vi "Main_Steuerung.vi"() -> ()   [LabVIEW 2016]
uses:
  <vilib>/rvi/interface/nirviReadWriteControl/nirviReadWriteControl.xnode
  NiFpgaLv.dll
  <vilib>/Utility/error.llb/Error Cluster From Error Code.vi
  <vilib>/rvi/interface/Simulation/niFpgaSimulationCallBeginRW.vi
  <vilib>/rvi/errors/niLvFpgaAdjustHostInterfaceError.vi
  <vilib>/rvi/interface/nirviOpenFPGA/nirviOpenFPGA.xnode
  <vilib>/rvi/interface/nirviMethod/nirviMethod.xnode
  <vilib>/FPGAPlugInAG/Dynamic/niLvFpga_Reset_Dynamic.vi
  <vilib>/FPGAPlugInAG/Dynamic/niLvFpga_Run_Dynamic.vi
  <vilib>/rvi/interface/nirviCloseFPGA/nirviCloseFPGA.xnode
  <vilib>/FPGAPlugInAG/Dynamic/niLvFpga_Abort_Dynamic.vi
  <vilib>/ptbypt/NI_PtbyPt.lvlib
  <vilib>/Analysis/NI_AALBase.lvlib
  <vilib>/Analysis/1siggen.llb/Ramp Pattern by Samples.vi
  <vilib>/regexp/Match Regular Expression.xnode
  <vilib>/FPGAPlugInAG/Dynamic/niLvFpga_Close_Dynamic.vi
  <vilib>/rvi/interface/common/dynamic/niFpgaDynamicAddResources.vi
  FPGA Bitfiles/AKZ1_FPGATarget_MainFPGA_-zWm+JuPuU4.lvbitx
  Main_FPGA.vi
  <vilib>/FPGAPlugInAG/cRIO-9082/niLvFpga_Open_cRIO-9082.vi
  FPGA Bitfiles/AKZ1_FPGATarget3_EncoderPosition&_wC3QGglG6Rs.lvbitx
  FPGA VIs/Encoder Position & Velocity (FPGA).vi
  <vilib>/FPGAPlugInAG/NI 9154/niLvFpga_Open_NI 9154.vi
panel:
  in  "Output Range Bremse L":T1={"output high"=10.0, "output low"=-10.0}
  in  "Output Range Bremse R":T1={"output high"=10.0, "output low"=-10.0}
  in  "Stop":bool
  in  "Systemreset / ON":bool
  out "Alarme":T2
  in  "Alarme On":T3={"A 1"=TRUE, "A 2"=TRUE, "A 3"=FALSE, "A 4"=TRUE, "A 5"=TRUE, "A 6"=TRUE, "A 7"=TRUE, "A 8"=TRUE, "A 9"=TRUE, "A 10"=TRUE, "A 11"=TRUE, "A 12"=TRUE, "A 13"=TRUE, "A 14"=TRUE, "A 15"=TRUE, "A 16"=TRUE, "A 17"=FALSE, "A 18"=FALSE, "A 19"=FALSE, "A 20"=FALSE, "A 21"=FALSE, "A 22"=FALSE, "A 23"=FALSE, "A 24"=FALSE}
  in  "Masteralarm On":bool
  out "Masteralarm":bool
  in  "PID gains Bremse L":T4={"proportional gain (Kc)"=5.0, "integral gain (Kc*Ts/Ti)"=0.1015625, "derivative gain (Kc*Td/Ts)"=0.0}
  in  "PID gains Bremse R":T4={"proportional gain (Kc)"=5.0, "integral gain (Kc*Ts/Ti)"=0.1015625, "derivative gain (Kc*Td/Ts)"=0.0}
  in  "PID gains Bremse H":T4={"proportional gain (Kc)"=5.0, "integral gain (Kc*Ts/Ti)"=0.1015625, "derivative gain (Kc*Td/Ts)"=0.0}
  in  "PID gains Fahrhebelsteller":T4={"proportional gain (Kc)"=1.5, "integral gain (Kc*Ts/Ti)"=0.1015625, "derivative gain (Kc*Td/Ts)"=0.0}
  out "Recht":dbl(knob) scale=-10.0..10.0
  out "Link":dbl(knob) scale=-10.0..10.0
  out "L":dbl
  out "R":dbl
  in  "Rampe Down":u32=5
  in  "Count (mSec) Rampe H":u32=2
  in  "Count (mSec) H":u32=10
  out "output Rampe H":dbl
  in  "milliseconds to wait Rampe H":u32=10
  in  "type Rampe H":u16(ring) items=["Linear", "Logarithmic"]
  in  "sample length H":i32=100
  in  "milliseconds to wait Fahrhebel":u32=10
  in  "type Fahrhebel":u16(ring) items=["Linear", "Logarithmic"]
  out "output Fahrhebel":dbl
  in  "Count (mSec) Fahrhebel":u32=22
  in  "sample length LR":i32=100
  in  "sample length DM":i32=100
  in  "Count (mSec) Normal LR":u32=10
  in  "type Rampe LR":u16(ring) items=["Linear", "Logarithmic"]
  out "output Rampe LR":dbl format="%.2f"
  in  "milliseconds to wait Rampe LR":u32=10
  in  "Count (mSec) Rampe LR":u32=2
  in  "error in (no error)":errorcluster
  out "Punktenanzahl":i32
  out "Punktentabelle":dbl[][](array[numeric])
  out "error out":errorcluster
  in  "Tab Control":enum32{"H", "L-R", "H-L-R", "System"}(tab)
  in  "PID Out H":bool=TRUE
  in  "Rout H":bool
  out "Wellendrehmoment mit Übersetzung  H":dbl(knob) scale=-2000.0..2000.0
  out "Drehmoment Hinten":dbl(knob) scale=-2000.0..2000.0
  out "Drehzahl Hinten":dbl(knob) scale=0.0..8000.0
  in  "Bremse\nFrei H":bool
  in  "Reset / On\n H":bool
  in  "Steuerung\nOn H":bool
  in  "Lüftung\nOn H":bool
  out "Meldungen H":T5
  in  "Wellendrehzahl\n Soll H":dbl(slide) scale=-8000.0..8000.0
  out "Wellendrehzahl mit Übersetzung H":dbl(knob) scale=0.0..12000.0
  in  "Übersetzung H":dbl=3.15
  in  "Start Rampe H":dbl=900.0
  in  "Ende Rampe H":dbl=5100.0
  in  "Zeit (Sec) Rampe H":i32=30
  out "Rampe H Aktiv":bool
  in  "Rampe H Stop":bool
  in  "Rampe H Start":bool
  in  "Übersetzung H\nmit":bool=TRUE
  out "Rampe H  LED":bool
  out "Startwert Rampe LR 2":dbl format="%#_3f"
  in  "Wellen\nmoment\n Soll H":dbl(slide) scale=-2000.0..2000.0
  in  "Drehzahl/moment H":bool
  in  "Rampe H Runter":bool
  in  "PID Out LR":bool=TRUE
  out "Startwert Rampe LR":dbl format="%#_3f"
  out "Rampe LR  LED":bool
  in  "Übersetzung LR\nmit":bool=TRUE
  out "Abweichung":dbl(knob) scale=-30.0..30.0
  in  "Wellen\nmoment\n Soll LR":dbl(slide) scale=-2000.0..2000.0
  in  "Drehzahl/moment LR":bool
  out "Wellendrehmoment mit Übersetzung":dbl(knob) scale=-400.0..400.0
  out "Drehmoment Rechts":dbl(knob) scale=-2000.0..2000.0
  out "Drehmoment Links":dbl(knob) scale=-2000.0..2000.0
  out "Drehzahl Rechts":dbl(knob) scale=-3000.0..3000.0
  out "Drehzahl Links":dbl(knob) scale=-3000.0..3000.0
  in  "Bremse\nFrei":bool
  in  "Reset / On":bool
  in  "Steuerung\nOn":bool
  in  "Lüftung\nOn":bool
  out "Meldungen L-R":T6
  in  "Wellen\ndrehzahl\n Soll":dbl(slide) scale=-3000.0..3000.0 scale format="%4d"
  out "Wellendrehzahl mit Übersetzung":dbl(knob) scale=0.0..5000.0
  in  "Übersetzung LR":dbl=3.88
  in  "Rampe LR Start":bool
  in  "Rampe LR Runter":bool
  in  "Rampe LR Stop":bool
  out "Rampe LR Aktiv":bool
  in  "Zeit (Sec) Rampe LR":i32=60
  in  "Ende Rampe LR":dbl=4800.0
  in  "Start Rampe LR":dbl=880.0
  in  "Rout LR":bool
  in  "Tab Control 2":enum32{"Benzinmotor", "Elektromototr"}(tab)
  out "Rampe Fahrregler  LED":bool
  in  "Fahrregler Runter":bool
  in  "Fahrregler Stop":bool
  out "Fahrregler Aktiv":bool
  in  "Fahrregler Start":bool
  in  "PID Regler Fahrhebel\nWellenmoment Soll":bool
  in  "Motor\nStart":bool
  in  "Vorglühen\nOn":bool
  in  "Zündung\nOn":bool
  in  "Kraftstoff\nOn":bool
  out "Fahrhebelsteller":u8(slide) scale=0.0..100.0
  in  "Fahrhebelsteller Soll":dbl(slide) scale=0.0..100.0
  in  "Freigabe Fahrhebel":bool
  in  "Kupplung\nOffen":bool=TRUE
  out "Kupplung":cluster{"Offen":bool, "Geschlossen":bool}
  in  "Zeit (Sec) Fahrregler":i32=20
  in  "Ende Fahrregler":dbl=100.0
  in  "Start Fahrregler":dbl
  in  "Kennfeld Wellenmoment laden\nx,xx Prozent einstellen":bool
  in  "Prozent":dbl=0.5
  in  "Temperaturregelung\nFreigabe":bool
  in  "Temperaturregelung\nWait":bool
  out "Höhe M":fxp<+/-,24,5> format="%#.2g"
  out "Endlage Unten M":bool
  out "Endlage Oben M":bool
  out "Oben M":bool
  out "Unten M":bool
  in  "Freigabe Höhe M":bool
  in  "Richtung Höhe M":bool
  in  "Freigabe Drehzahl M":bool
  in  "Richtung Drehzahl M":bool
  in  "Freigabe Bremse M":bool
  in  "Run Button":bool
  in  "Hydraulikpumpensteller":dbl=11.0
  in  "Manual":bool
  in  "Up Button":bool
  in  "Down Button":bool
  in  "RPMK":dbl=300.0
  in  "Drehmoment Motor":dbl
  in  "Hydraulikkupplung":dbl
  # "ohne"
  # "ohne"
  # "Links"
  # "Rechts"
  # "System nicht bereit!"
  # "Geschlossen"
  # "%"
  # "%"
  # "%"
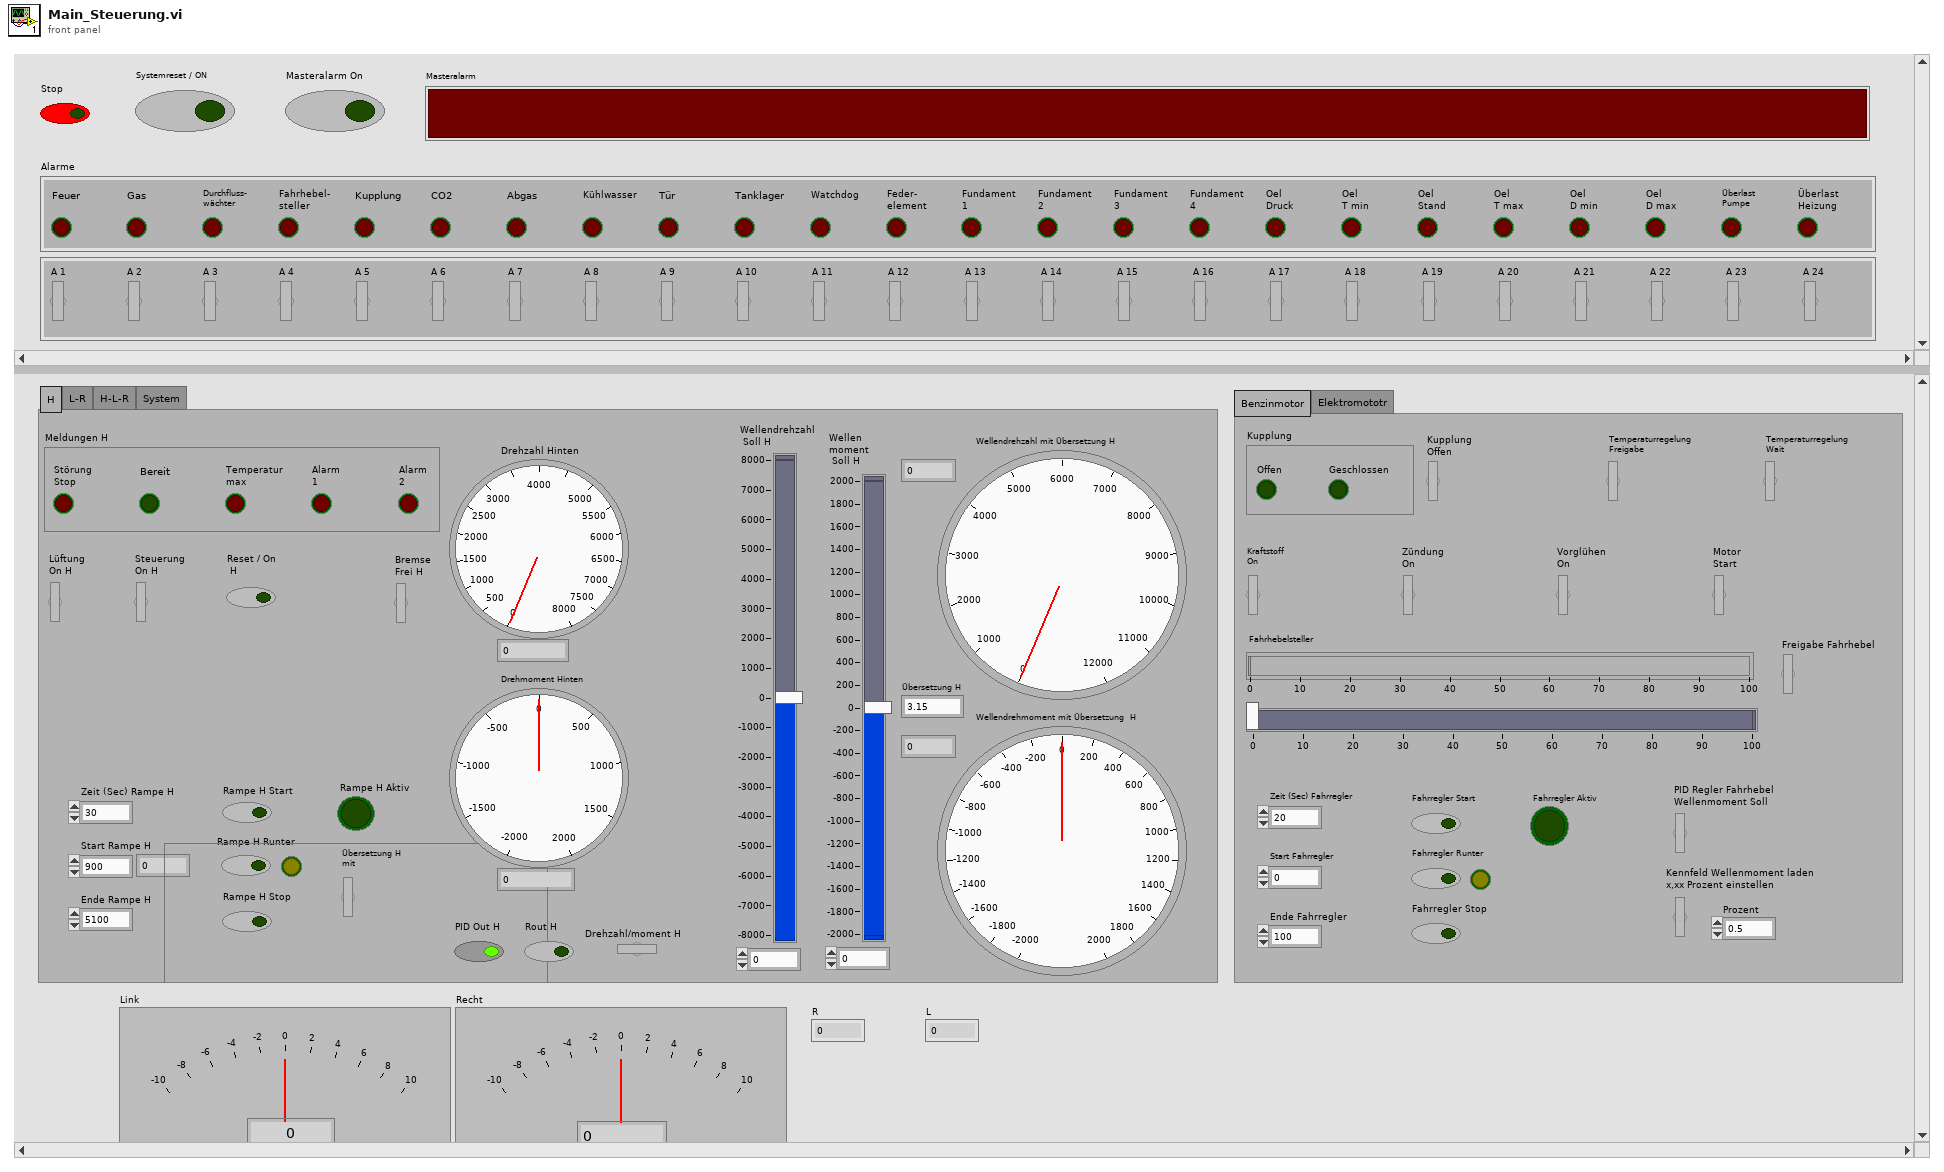
[diagram p1: front panel]
types:
  T1 = cluster{"output high":fxp<+/-,16,5>, "output low":fxp<+/-,16,5>}
  T2 = cluster{"Feuer\n":bool, "Gas\n":bool, "Durchfluss-\nwächter":bool, "Fahrhebel-\nsteller":bool, "Kupplung\n":bool, "CO2\n":bool, "Abgas\n":bool, "Kühlwasser\n":bool, "Tür\n":bool, "Tanklager\n":bool, "Watchdog\n":bool, "Feder-\nelement":bool, "Fundament\n1":bool, "Fundament\n2":bool, "Fundament\n3":bool, "Fundament\n4":bool, "Oel\nDruck":bool, "Oel\nT min":bool, "Oel\nStand":bool, "Oel\nT max":bool, "Oel\nD min":bool, "Oel\nD max":bool, "Überlast\nPumpe":bool, "Überlast\nHeizung":bool}
  T3 = cluster{"A 1":bool, "A 2":bool, "A 3":bool, "A 4":bool, "A 5":bool, "A 6":bool, "A 7":bool, "A 8":bool, "A 9":bool, "A 10":bool, "A 11":bool, "A 12":bool, "A 13":bool, "A 14":bool, "A 15":bool, "A 16":bool, "A 17":bool, "A 18":bool, "A 19":bool, "A 20":bool, "A 21":bool, "A 22":bool, "A 23":bool, "A 24":bool}
  T4 = cluster{"proportional gain (Kc)":fxp<+/-,16,8>, "integral gain (Kc*Ts/Ti)":fxp<+/-,16,8>, "derivative gain (Kc*Td/Ts)":fxp<+/-,16,8>}
  T5 = cluster{"Störung\nStop":bool, "Bereit\n":bool, "Temperatur\nmax":bool, "Alarm\n1":bool, "Alarm\n2":bool}
  T6 = cluster{"Störung\nStop":bool, "Bereit\n":bool, "Temperatur\nmax":bool, "Alarm\n1":bool, "Alarm\n2":bool, "Störung\nStop":bool, "Bereit\n":bool, "Temperatur\nmax":bool, "Alarm\n1":bool, "Alarm\n2":bool}
  T7 = enum16{"open", "replace", "create", "open or create", "replace or create", "replace or create with confirmation"}
  T8 = cluster{"Mod5/Alarm 1 Feuer":void, "Mod5/Alarm 2 Gas":bool, "Mod5/Alarm 3 Durchflusswächter":void, "Mod5/Alarm 4 Fahrhebelsteller":void, "Mod5/Alarm 5 Kupplung":void, "Mod5/Alarm 6 CO2":bool, "Mod5/Alarm 7 Abgas":void, "Mod5/Alarm 8 Kühlwasser":void, "Mod5/Alarm 9 Tür":void, "Mod5/Alarm 10 Tanklager":void, "Mod5/Alarm 11 Watchdog":bool, "Mod5/Alarm 12 Federelement":void, "Mod5/Alarm 13 Fundament 1":bool, "Mod5/Alarm 14 Fundament 2":bool, "Mod5/Alarm 15 Fundament 3":bool, "Mod5/Alarm 16 Fundament 4":bool, "Mod6/Alarm 17 Differnzdruck Öl":void, "Mod6/Alarm 19 Temperatur Min ÖL":void, "Mod6/Alarm 18 Nivau Öl":void, "Mod6/Alarm 20 Temperatur Max Öl":void, "Mod6/Alarm 21 Druck Min Öl":void, "Mod6/Alarm 22 Druck Max Öl":void, "Mod6/Alarm 23 Überlast Pumpe Öl":void, "Mod6/Alarm 24 Überlast Heizung Öl":void}
  T9 = cluster{"Mod5/Störung Bremse L":void, "Mod5/Bereit Bremse L":void, "Mod5/Temperatur Bremse L":void, "Mod5/Alarm 1 Bremse L":void, "Mod5/Alarm 2 Bremse L":void, "Mod5/Störung Bremse R":void, "Mod5/Bereit Bremse R":void, "Mod5/Temperatur Bremse R":void, "Mod5/Alarm 1 Bremse R":void, "Mod5/Alarm 2 Bremse R":void}
  T10 = cluster{"Mod6/Störung Bremse H":void, "Mod6/Bereit Bremse H":void, "Mod6/Temperatur Bremse H":void, "Mod6/Alarm 1 Bremse H":void, "Mod6/Alarm 2 Bremse H":void}
  T11 = cluster{"Mod6/Kupplung Zu":void, "Mod6/Kupplung Auf":void}
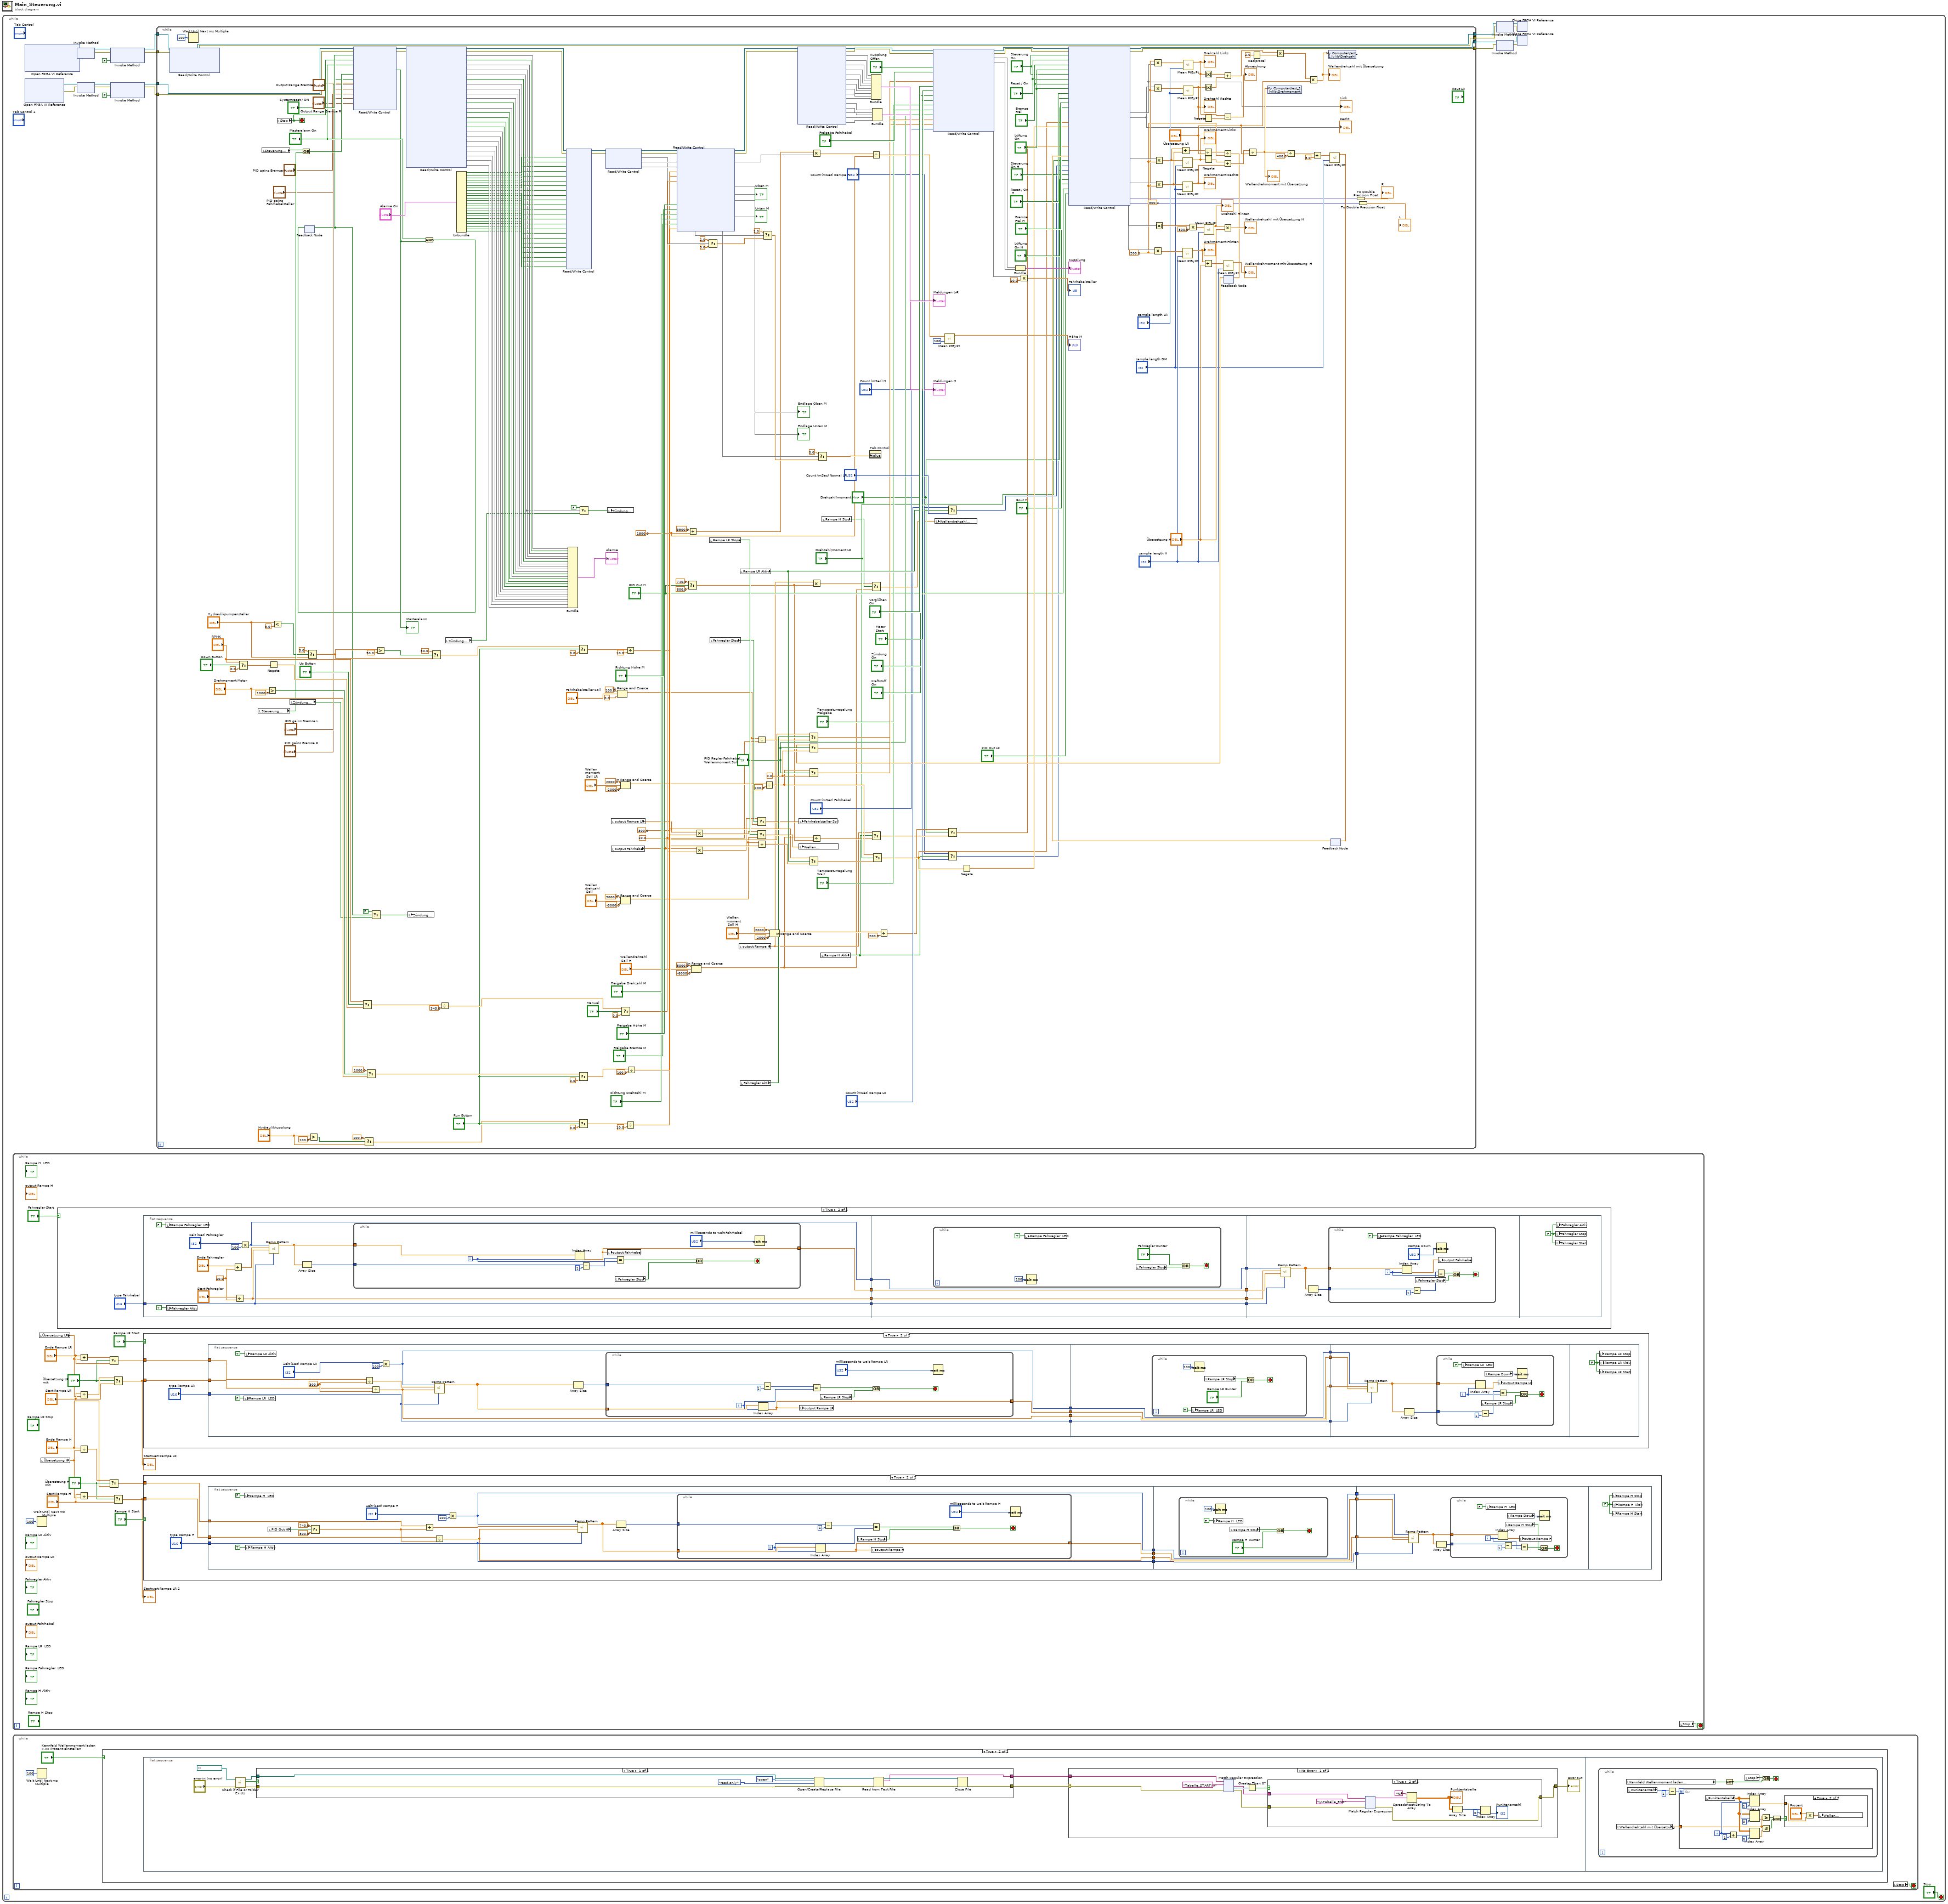
[diagram p0: block diagram]
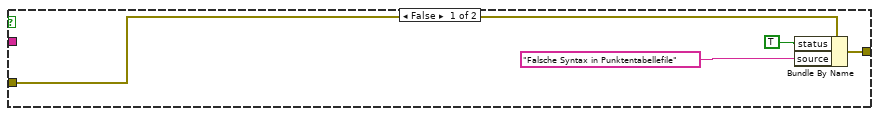
[diagram p3: hidden frame]
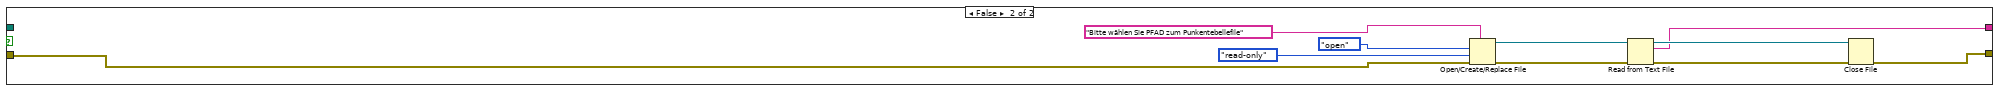
[diagram p5: hidden frame]
diagram:
  n1 = while {
    stop <- "Stop" stop-if-true
    n2 = while {
      stop <- w344 stop-if-true
      n3 = Wait Until Next ms Multiple(millisecond multiple=u32 100) -> ()  [unwired: 1 out]
      n4 = local read "Übersetzung LR"() -> (w336:dbl)
      n5 = local read "Übersetzung H"() -> (w328:dbl)
      n6 = case shown="True" "Fahrregler Start" {
        frame False {
        }
        frame True {
          n7 = flat-sequence {
            tunnel: "type Fahrhebel" -> [w426]
            tunnel: [w423] -> w418
            tunnel: [w426] -> w416
            tunnel: [w425] -> w414
            tunnel: [w424] -> w412
            tunnel: w418 -> [w447]
            tunnel: [w447] -> w417
            tunnel: w416 -> [w446]
            tunnel: [w446] -> w415
            tunnel: w414 -> [w445]
            tunnel: [w445] -> w413
            tunnel: w412 -> [w444]
            tunnel: [w444] -> w411
            tunnel: w417 -> [w458]
            tunnel: w415 -> [w457]
            tunnel: w413 -> [w456]
            tunnel: w411 -> [w455]
            frame #0 {
              w430 = 10.0 ("y")
              n8 = local write "Rampe Fahrregler  LED"(FALSE) -> ()
              n9 = local write "Fahrregler Aktiv"(TRUE) -> ()
              n10 = Divide(x="Ende Fahrregler", y=w430) -> (x/y=w432:dbl)
              n11 = Divide(x="Start Fahrregler", y=w430) -> (x/y=w424:dbl)
              n12 = Multiply(x="Zeit (Sec) Fahrregler", y=100) -> (x*y=w423:i32)
              n13 = call-poly <vilib>:"Ramp Pattern.vi"("type"=w426, "start"=w424, "end"=w432, "samples"=w423) -> ("Ramp Pattern"=w428:dbl[])  [unwired: 6 in, 1 out]
              n14 = Array Size(array=w428) -> (size(s)=w427:i32)
              n15 = while {
                tunnel: w428 -> [w443]
                tunnel: w427 -> [w442]
                tunnel: [w434] -> w425
                i -> [w439]
                stop <- w437 stop-if-true
                n16 = Index Array(array=w443, index=w439) -> (element=w434:dbl)
                n17 = Subtract(x=w442, y=1) -> (x-y=w440:i32)
                n18 = local write "output Fahrhebel"(w434) -> ()
                n19 = local read "Fahrregler Stop"() -> (w436:bool)
                n20 = Equal?(x=w440, y=w439) -> (x = y?=w438:bool)
                n21 = Or(x=w438, y=w436) -> (x .or. y?=w437:bool)
                n22 = Wait (ms)(milliseconds to wait="milliseconds to wait Fahrhebel") -> ()  [unwired: 1 out]
              }
            }
            frame #1 {
              n23 = while {
                stop <- w451 stop-if-true
                n24 = local write "Rampe Fahrregler  LED"(TRUE) -> ()
                n25 = Wait (ms)(milliseconds to wait=u32 100) -> ()  [unwired: 1 out]
                n26 = local read "Fahrregler Stop"() -> (w450:bool)
                n27 = Or(x="Fahrregler Runter", y=w450) -> (x .or. y?=w451:bool)
              }
            }
            frame #2 {
              n28 = call-poly <vilib>:"Ramp Pattern.vi"("type"=w457, "start"=w456, "end"=w455, "samples"=w458) -> ("Ramp Pattern"=w454:dbl[])  [unwired: 6 in, 1 out]
              n29 = Array Size(array=w454) -> (size(s)=w453:i32)
              n30 = while {
                tunnel: w454 -> [w469]
                tunnel: w453 -> [w468]
                i -> [w465]
                stop <- w463 stop-if-true
                n31 = local write "Rampe Fahrregler  LED"(FALSE) -> ()
                n32 = Index Array(array=w469, index=w465) -> (element=w461:dbl)
                n33 = Subtract(x=w468, y=1) -> (x-y=w466:i32)
                n34 = local read "Fahrregler Stop"() -> (w462:bool)
                n35 = Equal?(x=w466, y=w465) -> (x = y?=w464:bool)
                n36 = Wait (ms)(milliseconds to wait="Rampe Down") -> ()  [unwired: 1 out]
                n37 = local write "output Fahrhebel"(w461) -> ()
                n38 = Or(x=w464, y=w462) -> (x .or. y?=w463:bool)
              }
            }
            frame #3 {
              w470 = FALSE
              n39 = local write "Fahrregler Stop"(w470) -> ()
              n40 = local write "Fahrregler Start"(w470) -> ()
              n41 = local write "Fahrregler Aktiv"(w470) -> ()
            }
          }
        }
      }
      n42 = Divide(x="Ende Rampe LR", y=w336) -> (x/y=w341:dbl)
      n43 = Divide(x="Start Rampe LR", y=w336) -> (x/y=w339:dbl)
      n44 = Divide(x="Ende Rampe H", y=w328) -> (x/y=w332:dbl)
      n45 = Divide(x="Start Rampe H", y=w328) -> (x/y=w333:dbl)
      n46 = Select(t=w341, s="Übersetzung LR\nmit", f="Ende Rampe LR") -> (s? t:f=w342:dbl)
      n47 = Select(t=w332, s="Übersetzung H\nmit", f="Ende Rampe H") -> (s? t:f=w327:dbl)
      n48 = Select(t=w339, s="Übersetzung LR\nmit", f="Start Rampe LR") -> (s? t:f=w335:dbl)
      "Startwert Rampe LR" <- w335
      n49 = Select(t=w333, s="Übersetzung H\nmit", f="Start Rampe H") -> (s? t:f=w326:dbl)
      "Startwert Rampe LR 2" <- w326
      n50 = case shown="True" "Rampe LR Start" {
        tunnel: w335 -> [_ w472]
        tunnel: w342 -> [_ w471]
        frame False {
        }
        frame True {
          n51 = flat-sequence {
            tunnel: [w487] -> w480
            tunnel: [w492] -> w478
            tunnel: [w491] -> w476
            tunnel: [w489] -> w474
            tunnel: "type Rampe LR" -> [w489]
            tunnel: w472 -> [w482]
            tunnel: w471 -> [w483]
            tunnel: [w509] -> w481
            tunnel: w480 -> [w509]
            tunnel: [w508] -> w479
            tunnel: w478 -> [w508]
            tunnel: [w507] -> w477
            tunnel: w476 -> [w507]
            tunnel: [w506] -> w475
            tunnel: w474 -> [w506]
            tunnel: w481 -> [w520]
            tunnel: w479 -> [w519]
            tunnel: w477 -> [w518]
            tunnel: w475 -> [w517]
            frame #0 {
              w488 = 300.0
              n52 = local write "Rampe LR  LED"(FALSE) -> ()
              n53 = local write "Rampe LR Aktiv"(TRUE) -> ()
              n54 = Divide(x=w483, y=w488) -> (x/y=w493:dbl)
              n55 = Divide(x=w482, y=w488) -> (x/y=w492:dbl)
              n56 = Multiply(x="Zeit (Sec) Rampe LR", y=100) -> (x*y=w487:i32)
              n57 = call-poly <vilib>:"Ramp Pattern.vi"("type"=w489, "start"=w492, "end"=w493, "samples"=w487) -> ("Ramp Pattern"=w494:dbl[])  [unwired: 6 in, 1 out]
              n58 = Array Size(array=w494) -> (size(s)=w495:i32)
              n59 = while {
                tunnel: w494 -> [w505]
                tunnel: w495 -> [w504]
                tunnel: [w496] -> w491
                i -> [w501]
                stop <- w498 stop-if-true
                n60 = Index Array(array=w505, index=w501) -> (element=w496:dbl)
                n61 = Subtract(x=w504, y=1) -> (x-y=w502:i32)
                n62 = local write "output Rampe LR"(w496) -> ()
                n63 = Equal?(x=w502, y=w501) -> (x = y?=w500:bool)
                n64 = local read "Rampe LR Stop"() -> (w497:bool)
                n65 = Or(x=w500, y=w497) -> (x .or. y?=w498:bool)
                n66 = Wait (ms)(milliseconds to wait="milliseconds to wait Rampe LR") -> ()  [unwired: 1 out]
              }
            }
            frame #1 {
              n67 = while {
                stop <- w512 stop-if-true
                n68 = local write "Rampe LR  LED"(TRUE) -> ()
                n69 = Wait (ms)(milliseconds to wait=u32 100) -> ()  [unwired: 1 out]
                n70 = local read "Rampe LR Stop"() -> (w511:bool)
                n71 = Or(x=w511, y="Rampe LR Runter") -> (x .or. y?=w512:bool)
              }
            }
            frame #2 {
              n72 = call-poly <vilib>:"Ramp Pattern.vi"("type"=w517, "start"=w518, "end"=w519, "samples"=w520) -> ("Ramp Pattern"=w516:dbl[])  [unwired: 6 in, 1 out]
              n73 = Array Size(array=w516) -> (size(s)=w515:i32)
              n74 = while {
                tunnel: w516 -> [w531]
                tunnel: w515 -> [w530]
                i -> [w527]
                stop <- w525 stop-if-true
                n75 = local write "Rampe LR  LED"(FALSE) -> ()
                n76 = Index Array(array=w531, index=w527) -> (element=w523:dbl)
                n77 = Subtract(x=w530, y=1) -> (x-y=w528:i32)
                n78 = local read "Rampe LR Stop"() -> (w524:bool)
                n79 = local read "Rampe Down"() -> (w521:u32)
                n80 = local write "output Rampe LR"(w523) -> ()
                n81 = Equal?(x=w528, y=w527) -> (x = y?=w526:bool)
                n82 = Wait (ms)(milliseconds to wait=w521) -> ()  [unwired: 1 out]
                n83 = Or(x=w526, y=w524) -> (x .or. y?=w525:bool)
              }
            }
            frame #3 {
              w532 = FALSE
              n84 = local write "Rampe LR Stop"(w532) -> ()
              n85 = local write "Rampe LR Start"(w532) -> ()
              n86 = local write "Rampe LR Aktiv"(w532) -> ()
            }
          }
        }
      }
      n87 = case shown="True" "Rampe H Start" {
        tunnel: w327 -> [_ w356]
        tunnel: w326 -> [_ w355]
        frame False {
        }
        frame True {
          n88 = flat-sequence {
            tunnel: w356 -> [w370]
            tunnel: w355 -> [w369]
            tunnel: "type Rampe H" -> [w364]
            tunnel: [w364] -> w353
            tunnel: [w363] -> w351
            tunnel: [w362] -> w349
            tunnel: [w361] -> w347
            tunnel: w353 -> [w387]
            tunnel: [w387] -> w352
            tunnel: w351 -> [w386]
            tunnel: [w386] -> w350
            tunnel: w349 -> [w385]
            tunnel: [w385] -> w348
            tunnel: w347 -> [w384]
            tunnel: [w384] -> w346
            tunnel: w352 -> [w396]
            tunnel: w350 -> [w395]
            tunnel: w348 -> [w394]
            tunnel: w346 -> [w393]
            frame #0 {
              n89 = local write "Rampe H  LED"(FALSE ("Rampe H  LED")) -> ()
              n90 = local write "Rampe H Aktiv"(TRUE ("Rampe H Aktiv")) -> ()
              n91 = local read "PID Out H"() -> (w357:bool)
              n92 = Select(t=740.0, s=w357, f=800.0 ("y")) -> (s? t:f=w358:dbl)
              n93 = Divide(x=w370, y=w358) -> (x/y=w371:dbl)
              n94 = Divide(x=w369, y=w358) -> (x/y=w362:dbl)
              n95 = Multiply(x="Zeit (Sec) Rampe H", y=100) -> (x*y=w363:i32)
              n96 = call-poly <vilib>:"Ramp Pattern.vi"("type"=w364, "start"=w362, "end"=w371, "samples"=w363) -> ("Ramp Pattern"=w366:dbl[])  [unwired: 6 in, 1 out]
              n97 = Array Size(array=w366) -> (size(s)=w365:i32)
              n98 = while {
                tunnel: w366 -> [w382]
                tunnel: w365 -> [w381]
                tunnel: [w374] -> w361
                i -> [w379]
                stop <- w376 stop-if-true
                n99 = Index Array(array=w382, index=w379) -> (element=w374:dbl)
                n100 = Subtract(x=w381, y=1) -> (x-y=w378:i32)
                n101 = local read "Rampe H Stop"() -> (w375:bool)
                n102 = Equal?(x=w378, y=w379) -> (x = y?=w377:bool)
                n103 = local write "output Rampe H"(w374) -> ()
                n104 = Or(x=w377, y=w375) -> (x .or. y?=w376:bool)
                n105 = Wait (ms)(milliseconds to wait="milliseconds to wait Rampe H") -> ()  [unwired: 1 out]
              }
            }
            frame #1 {
              n106 = while {
                stop <- w390 stop-if-true
                n107 = local write "Rampe H  LED"(TRUE) -> ()
                n108 = Wait (ms)(milliseconds to wait=u32 100) -> ()  [unwired: 1 out]
                n109 = local read "Rampe H Stop"() -> (w389:bool)
                n110 = Or(x=w389, y="Rampe H Runter") -> (x .or. y?=w390:bool)
              }
            }
            frame #2 {
              n111 = call-poly <vilib>:"Ramp Pattern.vi"("type"=w396, "start"=w393, "end"=w394, "samples"=w395) -> ("Ramp Pattern"=w397:dbl[])  [unwired: 6 in, 1 out]
              n112 = Array Size(array=w397) -> (size(s)=w398:i32)
              n113 = while {
                tunnel: w397 -> [w409]
                tunnel: w398 -> [w408]
                i -> [w405]
                stop <- w403 stop-if-true
                n114 = local write "Rampe H  LED"(FALSE) -> ()
                n115 = Index Array(array=w409, index=w405) -> (element=w401:dbl)
                n116 = Subtract(x=w408, y=1) -> (x-y=w406:i32)
                n117 = local read "Rampe H Stop"() -> (w402:bool)
                n118 = local read "Rampe Down"() -> (w399:u32)
                n119 = local write "output Rampe H"(w401) -> ()
                n120 = Equal?(x=w406, y=w405) -> (x = y?=w404:bool)
                n121 = Or(x=w404, y=w402) -> (x .or. y?=w403:bool)
                n122 = Wait (ms)(milliseconds to wait=w399) -> ()  [unwired: 1 out]
              }
            }
            frame #3 {
              w410 = FALSE
              n123 = local write "Rampe H Stop"(w410) -> ()
              n124 = local write "Rampe H Start"(w410) -> ()
              n125 = local write "Rampe H Aktiv"(w410) -> ()
            }
          }
        }
      }
      n126 = local read "Stop"() -> (w344:bool)
    }
    n127 = while {
      stop <- w25 stop-if-true
      n128 = Wait Until Next ms Multiple(millisecond multiple=u32 100) -> ()  [unwired: 1 out]
      n129 = case shown="True" "Kennfeld Wellenmoment laden\nx,xx Prozent einstellen" {
        frame False {
        }
        frame True {
          n130 = flat-sequence {
            frame #0 {
              n131 = call <vilib>:"Check if File or Folder Exists.vi"("error in (no error)"="error in (no error)", "path"=path "") -> ("error out"=w31:errorcluster, "file or folder exists?"=w29:bool, "dup path"=w30:path)  [unwired: 7 in]
              n132 = case shown="True" w29 {
                tunnel: w30 -> [w289 _]
                tunnel: [w282 w293] -> w32
                tunnel: w31 -> [w281 w291]
                tunnel: [w280 w290] -> w33
                frame True {
                  n133 = Open/Create/Replace File(file path (use dialog)=w289, error in=w281, operation (0:open)=T7."open", access (0:read/write)=enum16{"read/write", "read-only", "write-only"}."read-only") -> (refnum out=w286:refnum<file>, error out=w285:errorcluster)  [unwired: 2 in, 1 out]
                  n134 = Read from Text File(file (use dialog)=w286, error in=w285) -> (refnum out=w283:refnum<file>, text=w282:string, error out=w284:errorcluster)  [unwired: 2 in, 1 out]
                  n135 = Close File(refnum=w283, error in=w284) -> (error out=w280:errorcluster)  [unwired: 1 out]
                }
                frame False {
                  n136 = Open/Create/Replace File(error in=w291, prompt="Bitte wählen Sie PFAD zum Punkentebellefile", operation (0:open)=T7."open", access (0:read/write)=enum16{"read/write", "read-only", "write-only"}."read-only") -> (refnum out=w297:refnum<file>, error out=w296:errorcluster)  [unwired: 2 in, 1 out]
                  n137 = Read from Text File(file (use dialog)=w297, error in=w296) -> (refnum out=w294:refnum<file>, text=w293:string, error out=w295:errorcluster)  [unwired: 2 in, 1 out]
                  n138 = Close File(refnum=w294, error in=w295) -> (error out=w290:errorcluster)  [unwired: 1 out]
                }
              }
              n139 = case shown="No Error" w33 {
                selector: w33 -> [w37 w279]
                tunnel: w32 -> [w42 _]
                tunnel: [w35 w279] -> w34
                frame No Error {
                  n140 = xnode "Match Regular Expression"("input string"=w42, "regular expression"="Tabelle_START\\n", "error in"=w37) -> ("after match"=w38:string, "offset past match"=w40:i32, "error out"=w36:errorcluster)  [unwired: 3 in, 2 out]
                  n141 = Greater Than 0?(x=w40) -> (x > 0?=w39:bool)
                  n142 = case shown="True" w39 {
                    tunnel: w38 -> [_ w56]
                    tunnel: w36 -> [w46 w54]
                    tunnel: [w43 w53] -> w35
                    frame False {
                      n143 = Bundle By Name(cluster=w46, "status"=TRUE, "source"="Falsche Syntax in Punktentabellefile") -> (w43:errorcluster)
                    }
                    frame True {
                      n144 = xnode "Match Regular Expression"("input string"=w56, "regular expression"="\\nTabelle_END", "error in"=w54) -> ("before match"=w52:string, "error out"=w53:errorcluster)  [unwired: 3 in, 3 out]
                      n145 = Spreadsheet String To Array(format string="%f", spreadsheet string=w52) -> (array=w47:dbl[][])  [unwired: 2 in]
                      "Punktentabelle" <- w47
                      n146 = Array Size(array=w47) -> (size(s)=w50:i32[])
                      n147 = Index Array(array=w50, index=0) -> (element=→"Punktenanzahl":i32)
                    }
                  }
                }
                frame Error {
                }
              }
              "error out" <- w34
            }
            frame #1 {
              n148 = while {
                stop <- w302 stop-if-true
                n149 = local read "Wellendrehzahl mit Übersetzung"() -> (w301:dbl)
                n150 = local read "Kennfeld Wellenmoment laden\nx,xx Prozent einstellen"() -> (w303:bool)
                n151 = local read "Punktenanzahl"() -> (w306:i32)
                n152 = Subtract(x=w306, y=1) -> (x-y=w305:i32)
                n153 = for {
                  N: w305 -> [_]
                  tunnel: w301 -> [w308]
                  i -> [w318]
                  n154 = local read "Punktentabelle"() -> (w314:dbl[][])
                  n155 = Add(x=w318, y=1) -> (x+y=w315:i32)
                  n156 = Index Array(array=w314, index (row)=w318, index (col)=1 ("Deaktivierter Index (Spalte)")) -> (element=w320:dbl)
                  n157 = Index Array(array=w314, index (row)=w318, index (col)=0 ("Index (Spalte)")) -> (element=w309:dbl)
                  n158 = Index Array(array=w314, index (row)=w315, index (col)=0 ("Index (Spalte)")) -> (element=w310:dbl)
                  n159 = Greater Or Equal?(x=w308, y=w309) -> (x >= y?=w313:bool)
                  n160 = Less Or Equal?(x=w308, y=w310) -> (x <= y?=w312:bool)
                  n161 = And(x=w313, y=w312) -> (x .and. y?=w311:bool)
                  n162 = case shown="True" w311 {
                    tunnel: w320 -> [_ w324]
                    frame False {
                    }
                    frame True {
                      n163 = Multiply(x="Prozent", y=w324) -> (x*y=w323:dbl)
                      n164 = local write "Wellen\nmoment\n Soll LR"(w323) -> ()
                    }
                  }
                }
                n165 = Not(x=w303) -> (.not. x?=w300:bool)
                n166 = local read "Stop"() -> (w304:bool)
                n167 = Or(x=w304, y=w300) -> (x .or. y?=w302:bool)
              }
            }
          }
        }
      }
      n168 = local read "Stop"() -> (w25:bool)
    }
    n169 = xnode "Open FPGA VI Reference"() -> ("FPGA VI Reference Out"=w11:refnum<k20>, "error out"=w10:errorcluster)  [unwired: 2 in]
    n170 = xnode "Open FPGA VI Reference"() -> ("FPGA VI Reference Out"=w19:refnum<k20>, "error out"=w18:errorcluster)  [unwired: 2 in]
    n171 = xnode "Invoke Method"("FPGA VI Reference In"=w11, "error in"=w10) -> ("FPGA VI Reference Out"=w9:refnum<k20>, "error out"=w8:errorcluster)
    n172 = xnode "Invoke Method"("FPGA VI Reference In"=w19, "error in"=w18) -> ("FPGA VI Reference Out"=w17:refnum<k20>, "error out"=w16:errorcluster)
    n173 = xnode "Invoke Method"("FPGA VI Reference In"=w9, "error in"=w8, "Wait Until Done (F)"=FALSE) -> ("FPGA VI Reference Out"=w6:refnum<k20>, "error out"=w5:errorcluster)
    n174 = xnode "Invoke Method"("FPGA VI Reference In"=w17, "error in"=w16, "Wait Until Done (F)"=FALSE) -> ("FPGA VI Reference Out"=w12:refnum<k20>, "error out"=w23:errorcluster)
    n175 = while {
      tunnel: w12 -> [w860]
      tunnel: w23 -> [w859]
      tunnel: [w666] -> w22
      tunnel: [w704] -> w20
      tunnel: w6 -> [w575]
      tunnel: w5 -> [w574]
      tunnel: [w573] -> w2
      tunnel: [w572] -> w1
      stop <- w806 stop-if-true
      w587 = 10.0 ("f")
      w561 = 300.0 ("y")
      w636 = 0.0 ("f")
      w745 = 1800.0 ("y")
      w620 = 200.0 ("y")
      w645 = 300.0 ("x")
      n176 = xnode "Read/Write Control"("FPGA VI Reference In"=w575, "error in"=w574) -> ("FPGA VI Reference Out"=w573:refnum<k20>, "error out"=w572:errorcluster)  [unwired: 1 in, 3 out]
      n177 = Wait Until Next ms Multiple(millisecond multiple=u32 100) -> ()  [unwired: 1 out]
      n178 = Select(t="RPMK", s="Down Button", f=0.0) -> (s? t:f=w736:dbl)
      n179 = local read "Steuerung\nOn H"() -> (w680:bool)
      n180 = local read "Steuerung\nOn"() -> (w679:bool)
      n181 = Greater?(x="Drehmoment Motor", y=1000.0) -> (0:w717:bool)
      n182 = Negate(x=w736) -> (-x=w734:dbl)
      n183 = Less?(x="Hydraulikpumpensteller", y=5.0) -> (x < y?=w663:bool)
      n184 = local read "Stop"() -> (w806:bool)
      n185 = local read "Zündung\nOn"() -> (w613:bool)
      n186 = Or(x=w679, y=w680) -> (x .or. y?=w678:bool)
      n187 = feedback #1() -> (w616:bool)  [unwired: 1 in]
      n188 = Select(t=5.0, s=w663, f="Hydraulikpumpensteller") -> (s? t:f=w660:dbl)
      n189 = Greater?(x="Hydraulikkupplung", y=100.0) -> (0:w675:bool)
      n190 = xnode "Read/Write Control"("FPGA VI Reference In"=w860, "error in"=w859, "Mod3/Systemreset/ON"="Systemreset / ON", "stop"=w806, "Alarm On"="Masteralarm On", "Mod3/Blitzlicht"=w678, "Mod3/Horn"=w616, "PID gains Bremse L"="PID gains Bremse L", "PID gains Bremse R"="PID gains Bremse R", "PID gains Bremse H"="PID gains Bremse H", "PID gains"="PID gains Fahrhebelsteller", "Output Range Bremse R"="Output Range Bremse R", "Output Range Bremse L"="Output Range Bremse L") -> ("FPGA VI Reference Out"=w858:refnum<k20>, "error out"=w759:errorcluster, "Alarm"=w774:bool)
      "Masteralarm" <- w774
      n191 = Select(t="RPMK", s="Up Button", f=w734) -> (s? t:f=w733:dbl)
      n192 = Select(t=100.0, s=w675, f="Hydraulikkupplung") -> (s? t:f=w671:dbl)
      n193 = Select(t=1000.0, s=w717, f="Drehmoment Motor") -> (s? t:f=w714:dbl)
      n194 = Select(t=FALSE, s=w616, f=w613) -> (s? t:f=w615:bool)
      n195 = Greater?(x=w660, y=50.0) -> (0:w728:bool)
      n196 = xnode "Read/Write Control"("FPGA VI Reference In"=w858, "error in"=w759) -> ("FPGA VI Reference Out"=w857:refnum<k20>, "error out"=w710:errorcluster, "Mod5/Alarm 1 Feuer"=w856, "Mod5/Alarm 2 Gas"=w855:bool, "Mod5/Alarm 3 Durchflusswächter"=w853, "Mod5/Alarm 4 Fahrhebelsteller"=w607, "Mod5/Alarm 5 Kupplung"=w852, "Mod5/Alarm 6 CO2"=w851:bool, "Mod5/Alarm 7 Abgas"=w850, "Mod5/Alarm 8 Kühlwasser"=w849, "Mod5/Alarm 9 Tür"=w848, "Mod5/Alarm 10 Tanklager"=w847, "Mod5/Alarm 11 Watchdog"=w846:bool, "Mod5/Alarm 12 Federelement"=w845, "Mod5/Alarm 13 Fundament 1"=w844:bool, "Mod5/Alarm 14 Fundament 2"=w843:bool, "Mod5/Alarm 15 Fundament 3"=w842:bool, "Mod5/Alarm 16 Fundament 4"=w841:bool, "Mod6/Alarm 17 Differnzdruck Öl"=w840, "Mod6/Alarm 19 Temperatur Min ÖL"=w839, "Mod6/Alarm 18 Nivau Öl"=w838, "Mod6/Alarm 20 Temperatur Max Öl"=w837, "Mod6/Alarm 21 Druck Min Öl"=w836, "Mod6/Alarm 22 Druck Max Öl"=w835, "Mod6/Alarm 23 Überlast Pumpe Öl"=w834, "Mod6/Alarm 24 Überlast Heizung Öl"=w833)
      n197 = local write "Zündung\nOn"(w615) -> ()
      n198 = And(x="Masteralarm On", y=w774) -> (x .and. y?=w773:bool)
      n199 = feedback-in #1(w773) -> ()
      n200 = Select(t=50.0, s=w728, f=w660) -> (s? t:f=w676:dbl)
      n201 = Divide(x=w733, y=345.0) -> (x/y=w731:dbl)
      n202 = local read "Zündung\nOn"() -> (w610:bool)
      n203 = Unbundle("Alarme On") -> ("A 1"=w830:bool, "A 2"=w829:bool, "A 3"=w828:bool, "A 4"=w827:bool, "A 5"=w826:bool, "A 6"=w825:bool, "A 7"=w824:bool, "A 8"=w823:bool, "A 9"=w822:bool, "A 10"=w821:bool, "A 11"=w820:bool, "A 12"=w819:bool, "A 13"=w818:bool, "A 14"=w817:bool, "A 15"=w816:bool, "A 16"=w815:bool, "A 17"=w814:bool, "A 18"=w813:bool, "A 19"=w812:bool, "A 20"=w811:bool, "A 21"=w810:bool, "A 22"=w809:bool, "A 23"=w808:bool, "A 24"=w807:bool)
      n204 = xnode "Read/Write Control"("FPGA VI Reference In"=w857, "error in"=w710, "Alarm 1 On"=w830, "Alarm 2 On"=w829, "Alarm 3 On"=w828, "Alarm 4 On"=w827, "Alarm 5 On"=w826, "Alarm 6 On"=w825, "Alarm 7 On"=w824, "Alarm 8 On"=w823, "Alarm 9 On"=w822, "Alarm 10 On"=w821, "Alarm 11 On"=w820, "Alarm 12 On"=w819, "Alarm 13 On"=w818, "Alarm 14 On"=w817, "Alarm 15 On"=w816, "Alarm 16 On"=w815, "Alarm 17 On"=w814, "Alarm 18 On"=w813, "Alarm 19 On"=w812, "Alarm 20 On"=w811, "Alarm 21 On"=w810, "Alarm 22 On"=w809, "Alarm 23 On"=w808, "Alarm 24 On"=w807) -> ("FPGA VI Reference Out"=w832:refnum<k20>, "error out"=w709:errorcluster)
      n205 = Bundle("Mod5/Alarm 1 Feuer"=w856, "Mod5/Alarm 2 Gas"=w855, "Mod5/Alarm 3 Durchflusswächter"=w853, "Mod5/Alarm 4 Fahrhebelsteller"=w607, "Mod5/Alarm 5 Kupplung"=w852, "Mod5/Alarm 6 CO2"=w851, "Mod5/Alarm 7 Abgas"=w850, "Mod5/Alarm 8 Kühlwasser"=w849, "Mod5/Alarm 9 Tür"=w848, "Mod5/Alarm 10 Tanklager"=w847, "Mod5/Alarm 11 Watchdog"=w846, "Mod5/Alarm 12 Federelement"=w845, "Mod5/Alarm 13 Fundament 1"=w844, "Mod5/Alarm 14 Fundament 2"=w843, "Mod5/Alarm 15 Fundament 3"=w842, "Mod5/Alarm 16 Fundament 4"=w841, "Mod6/Alarm 17 Differnzdruck Öl"=w840, "Mod6/Alarm 19 Temperatur Min ÖL"=w839, "Mod6/Alarm 18 Nivau Öl"=w838, "Mod6/Alarm 20 Temperatur Max Öl"=w837, "Mod6/Alarm 21 Druck Min Öl"=w836, "Mod6/Alarm 22 Druck Max Öl"=w835, "Mod6/Alarm 23 Überlast Pumpe Öl"=w834, "Mod6/Alarm 24 Überlast Heizung Öl"=w833) -> (→"Alarme":T8)  [unwired: 1 in]
      n206 = Select(t=w676, s="Run Button", f=0.0) -> (s? t:f=w741:dbl)
      n207 = Select(t=w714, s="Run Button", f=0.0) -> (s? t:f=w713:dbl)
      n208 = Select(t=w671, s="Run Button", f=0.0) -> (s? t:f=w670:dbl)
      n209 = Select(t=FALSE, s=w607, f=w610) -> (s? t:f=w608:bool)
      n210 = xnode "Read/Write Control"("FPGA VI Reference In"=w832, "error in"=w709) -> ("FPGA VI Reference Out"=w725:refnum<k20>, "error out"=w708:errorcluster, "Mod6/Anlage H-L-R"=w798, "Mod6/Anlage H"=w805, "Mod6/Anlage L-R"=w801)
      n211 = local write "Zündung\nOn"(w608) -> ()
      n212 = local read "output Rampe LR"() -> (w647:dbl)
      n213 = local read "output Fahrhebel"() -> (w626:dbl)
      n214 = In Range and Coerce(upper limit=100.0, x="Fahrhebelsteller Soll", lower limit=0.0) -> (coerced(x)=w585:dbl)  [unwired: 1 out]
      n215 = In Range and Coerce(upper limit=2000.0, x="Wellen\nmoment\n Soll LR", lower limit=-2000.0) -> (coerced(x)=w597:dbl)  [unwired: 1 out]
      n216 = In Range and Coerce(upper limit=3000.0, x="Wellen\ndrehzahl\n Soll", lower limit=-3000.0) -> (coerced(x)=w602:dbl)  [unwired: 1 out]
      n217 = Select(t=w731, s="Manual", f=0.0) -> (s? t:f=w726:dbl)
      n218 = Divide(x=w741, y=10.0) -> (x/y=w655:dbl)
      n219 = Divide(x=w670, y=10.0) -> (x/y=w668:dbl)
      n220 = Divide(x=w713, y=100.0) -> (x/y=w711:dbl)
      n221 = xnode "Read/Write Control"("FPGA VI Reference In"=w725, "error in"=w708, "Mod7/Hydraulikkupplung Soll"=w668, "Mod7/Hydraulikpumpensteller Soll"=w655, "Mod7/Höhe M Soll"=w726, "Mod4/Freigabe Höhe M"="Freigabe Höhe M", "Mod4/Richtung Höhe M"="Richtung Höhe M", "Mod4/Freigabe Drehzahl M"="Freigabe Drehzahl M", "Mod4/Richtung Drehzahl M"="Richtung Drehzahl M", "Mod4/Freigabe Bremse M"="Freigabe Bremse M", "Mod7/Drehmoment M Soll"=w711) -> ("FPGA VI Reference Out"=w758:refnum<k20>, "error out"=w707:errorcluster, "Mod8/Höhe M"=w747, "Mod6/Endlage Oben M"=→"Endlage Oben M", "Mod6/Oben M"=→"Oben M", "Mod6/Unten M"=→"Unten M", "Mod6/Endlage Unten M"=→"Endlage Unten M")  [unwired: 2 out]
      n222 = Select(t=740.0, s="PID Out H", f=800.0) -> (s? t:f=w551:dbl)
      n223 = Add(x=3900.0, y=w745) -> (x+y=w748:dbl)
      n224 = In Range and Coerce(upper limit=8000.0, x="Wellendrehzahl\n Soll H", lower limit=-8000.0) -> (coerced(x)=w549:dbl)  [unwired: 1 out]
      n225 = Multiply(x=w647, y=w645) -> (x*y=w646:dbl)
      n226 = Multiply(x=w626, y=w587) -> (x*y=w627:dbl)
      n227 = Select(t=2.0, s=w798, f=3.0) -> (s? t:f=w799:dbl)
      n228 = local read "Rampe LR Stop"() -> (w648:bool)
      n229 = local read "Fahrregler Stop"() -> (w629:bool)
      n230 = local read "output Rampe H"() -> (w552:dbl)
      n231 = local read "Rampe LR Aktiv"() -> (w651:bool)
      n232 = local read "Fahrregler Aktiv"() -> (w630:bool)
      n233 = Select(t=w627, s=w629, f=w585) -> (s? t:f=w628:dbl)
      n234 = Select(t=w646, s=w648, f=w602) -> (s? t:f=w649:dbl)
      n235 = Divide(x=w585, y=w587) -> (x/y=w625:dbl)
      n236 = Divide(x=w602, y=w645) -> (x/y=w654:dbl)
      n237 = Select(t=1.0, s=w801, f=w799) -> (s? t:f=w802:dbl)
      n238 = Divide(x=w597, y=200.0) -> (x/y=w604:dbl)
      n239 = In Range and Coerce(upper limit=2000.0, x="Wellen\nmoment\n Soll H", lower limit=-2000.0) -> (coerced(x)=w579:dbl)  [unwired: 1 out]
      n240 = xnode "Read/Write Control"("FPGA VI Reference In"=w758, "error in"=w707) -> ("FPGA VI Reference Out"=w795:refnum<k20>, "error out"=w706:errorcluster, "Mod5/Störung Bremse L"=w793, "Mod5/Bereit Bremse L"=w792, "Mod5/Temperatur Bremse L"=w791, "Mod5/Alarm 1 Bremse L"=w790, "Mod5/Alarm 2 Bremse L"=w789, "Mod5/Störung Bremse R"=w788, "Mod5/Bereit Bremse R"=w787, "Mod5/Temperatur Bremse R"=w786, "Mod5/Alarm 1 Bremse R"=w785, "Mod5/Alarm 2 Bremse R"=w784, "Mod6/Störung Bremse H"=w686, "Mod6/Bereit Bremse H"=w685, "Mod6/Temperatur Bremse H"=w684, "Mod6/Alarm 1 Bremse H"=w683, "Mod6/Alarm 2 Bremse H"=w682)
      n241 = local write "Fahrhebelsteller Soll"(w628) -> ()
      n242 = local write "Wellen\ndrehzahl\n Soll"(w649) -> ()
      n243 = Select(t=w626, s=w630, f=w625) -> (s? t:f=w631:dbl)
      n244 = Select(t=w604, s="PID Regler Fahrhebel\nWellenmoment Soll", f=w636) -> (s? t:f=w637:dbl)
      n245 = Select(t=w647, s=w651, f=w654) -> (s? t:f=w599:dbl)
      n246 = Multiply(x=w748, y=w747) -> (x*y=w746:dbl)
      n247 = Multiply(x=w552, y=w551) -> (x*y=w550:dbl)
      n248 = Divide(x=w549, y=w551) -> (x/y=w558:dbl)
      n249 = Select(t=0.0, s=w805, f=w802) -> (s? t:f=w804:dbl)
      n250 = local read "Rampe H Aktiv"() -> (w556:bool)
      n251 = local read "Rampe H Stop"() -> (w547:bool)
      n252 = property on="Tab Control" class="TabCtl (strict)"("Value"=w804) -> ()  [unwired: 2 in, 2 out]
      n253 = Bundle("Mod5/Störung Bremse L"=w793, "Mod5/Bereit Bremse L"=w792, "Mod5/Temperatur Bremse L"=w791, "Mod5/Alarm 1 Bremse L"=w790, "Mod5/Alarm 2 Bremse L"=w789, "Mod5/Störung Bremse R"=w788, "Mod5/Bereit Bremse R"=w787, "Mod5/Temperatur Bremse R"=w786, "Mod5/Alarm 1 Bremse R"=w785, "Mod5/Alarm 2 Bremse R"=w784) -> (→"Meldungen L-R":T9)  [unwired: 1 in]
      n254 = Divide(x=w746, y=w745) -> (x/y=w743:dbl)
      n255 = Select(t=w550, s=w547, f=w549) -> (s? t:f=w548:dbl)
      n256 = Select(t=w552, s=w556, f=w558) -> (s? t:f=w557:dbl)
      n257 = Bundle("Mod6/Störung Bremse H"=w686, "Mod6/Bereit Bremse H"=w685, "Mod6/Temperatur Bremse H"=w684, "Mod6/Alarm 1 Bremse H"=w683, "Mod6/Alarm 2 Bremse H"=w682) -> (→"Meldungen H":T10)  [unwired: 1 in]
      n258 = Select(t=w604, s="Drehzahl/moment LR", f=w599) -> (s? t:f=w605:dbl)
      n259 = Divide(x=w579, y=200.0) -> (x/y=w577:dbl)
      n260 = local write "Wellendrehzahl\n Soll H"(w548) -> ()
      n261 = call <vilib>:"Mean PtByPt.vi"("x"=w743, "sample length"=100) -> ("mean"=→"Höhe M":dbl)  [unwired: 2 in, 1 out]
      n262 = Select(t="Count (mSec) Rampe LR", s=w651, f="Count (mSec) Normal LR") -> (s? t:f=w652:u32)
      n263 = Select(t=w577, s="Drehzahl/moment H", f=w557) -> (s? t:f=w576:dbl)
      n264 = Select(t="Count (mSec) Rampe H", s=w556, f="Count (mSec) H") -> (s? t:f=w553:u32)
      n265 = Negate(x=w605) -> (-x=w657:dbl)
      n266 = feedback #2() -> (w632:dbl)  [unwired: 1 in]
      n267 = Select(t=w632, s="PID Regler Fahrhebel\nWellenmoment Soll", f=w636) -> (s? t:f=w634:dbl)
      n268 = xnode "Read/Write Control"("FPGA VI Reference In"=w795, "error in"=w706, "Mod4/Kupplung"="Kupplung\nOffen", "Mod3/Fahrhebelsteller Freigabe"="Freigabe Fahrhebel", "Fahrhebelsteller Soll (%)"=w631, "Mod3/Motor Vorglühen On"="Vorglühen\nOn", "Mod3/Motor Start"="Motor\nStart", "Mod3/Motor Zündung On"="Zündung\nOn", "Mod3/Kraftstoffpumpe On"="Kraftstoff\nOn", "Mod4/Temperaturregelung Off"="Temperaturregelung\nWait", "Mod4/Temperaturregelung Freigabe"="Temperaturregelung\nFreigabe", "Regler Fahrhebelsteller"="PID Regler Fahrhebel\nWellenmoment Soll", "Vorgabe Fahrhebelsteller"=w637, "Ist Fahrhebelsteller"=w634, "Count (mSec) Fahrhebel"="Count (mSec) Fahrhebel") -> ("FPGA VI Reference Out"=w771:refnum<k20>, "error out"=w705:errorcluster, "Mod6/Kupplung Zu"=w769, "Mod6/Kupplung Auf"=w768, "Mod8/Fahrhebelsteller"=w760)
      n269 = Bundle("Mod6/Kupplung Zu"=w769, "Mod6/Kupplung Auf"=w768) -> (→"Kupplung":T11)  [unwired: 1 in]
      n270 = Multiply(x=w760, y=10.0) -> (x*y=→"Fahrhebelsteller":dbl)
      n271 = Reciprocal(x=2.0) -> (1/x=w779:dbl)
      n272 = feedback #3() -> (w722:dbl)  [unwired: 1 in]
      n273 = xnode "Read/Write Control"("FPGA VI Reference In"=w771, "error in"=w705, "Mod3/Steuerung On Bremse L"="Steuerung\nOn", "Mod3/Steuerungsreset Bremse L"="Reset / On", "Mod3/Bremsenfunktion On Bremse L"="Bremse\nFrei", "Mod3/Anlage On Bremse L"="Lüftung\nOn", "Mod3/Steuerung On Bremse R"="Steuerung\nOn", "Mod3/Steuerungsreset Bremse R"="Reset / On", "Mod3/Bremsenfunktion On Bremse R"="Bremse\nFrei", "Mod3/Anlage On Bremse R"="Lüftung\nOn", "Mod4/Steuerung On Bremse H"="Steuerung\nOn H", "Mod4/Steuerungsreset Bremse H"="Reset / On\n H", "Mod4/Bremsenfunktion On Bremse H"="Bremse\nFrei H", "Mod4/Anlage On Bremse H"="Lüftung\nOn H", "Vorgabe Bremse L"=w605, "Vorgabe Bremse R"=w657, "Vorgabe Bremse H"=w576, "Mod7/Out 1"=w722, "Drehzahl/moment LR"="Drehzahl/moment LR", "Count (mSec)"=w652, "Count (mSec) H"=w553, "Rout LR"="Drehzahl/moment LR", "Drehzahl/moment H"="Drehzahl/moment H", "Rout H"="Rout H", "PID Out H"="PID Out H", "PID Out LR"="PID Out LR") -> ("FPGA VI Reference Out"=w666:refnum<k20>, "error out"=w704:errorcluster, "Mod2/Drehzahl Bremse L"=w534, "Mod2/Drehzahl Bremse R"=w533, "Mod8/Drehmoment Bremse L"=w776, "Mod8/Drehmoment Bremse  R"=w592, "Mod2/Drehzahl Bremse H"=w697, "Mod8/Drehmoment Bremse H"=w691, "R"=w540:fxp<+/-,17,6>, "L"=w539:fxp<+/-,17,6>)
      "Link" <- w534
      "Recht" <- w533
      n274 = Multiply(x=w561, y=w534) -> (x*y=w640:dbl)
      n275 = Multiply(x=w533, y=w561) -> (x*y=w639:dbl)
      n276 = Multiply(x=w691, y=w620) -> (x*y=w692:dbl)
      n277 = Multiply(x=w776, y=w620) -> (x*y=w624:dbl)
      n278 = Multiply(x=w592, y=w620) -> (x*y=w623:dbl)
      n279 = Absolute Value(x=w697) -> (abs(x)=w696:dbl)
      n280 = Add(x=w624, y=w623) -> (x+y=w622:dbl)
      n281 = call <vilib>:"Mean PtByPt.vi"("x"=w624, "sample length"="sample length DM") -> ("mean"=w545:dbl)  [unwired: 2 in, 1 out]
      "Drehmoment Links" <- w545
      n282 = call <vilib>:"Mean PtByPt.vi"("x"=w623, "sample length"="sample length DM") -> ("mean"=w543:dbl)  [unwired: 2 in, 1 out]
      "Drehmoment Rechts" <- w543
      n283 = call <vilib>:"Mean PtByPt.vi"("x"=w692, "sample length"="sample length H") -> ("mean"=w688:dbl)  [unwired: 2 in, 1 out]
      "Drehmoment Hinten" <- w688
      n284 = call <vilib>:"Mean PtByPt.vi"("x"=w640, "sample length"="sample length LR") -> ("mean"=w563:dbl)  [unwired: 2 in, 1 out]
      "Drehzahl Links" <- w563
      n285 = call <vilib>:"Mean PtByPt.vi"("x"=w639, "sample length"="sample length LR") -> ("mean"=w562:dbl)  [unwired: 2 in, 1 out]
      "Drehzahl Rechts" <- w562
      n286 = Multiply(x=w696, y=800.0) -> (x*y=w695:dbl)
      n287 = Divide(x=w622, y="Übersetzung LR") -> (x/y=w621:dbl)
      n288 = Divide(x=w688, y="Übersetzung H") -> (x/y=w690:dbl)
      n289 = Absolute Value(x=w563) -> (abs(x)=w566:dbl)
      n290 = Absolute Value(x=w562) -> (abs(x)=w565:dbl)
      n291 = Negate(x=w562) -> (-x=w542:dbl)
      n292 = Negate(x=w545) -> (-x=w544:dbl)
      n293 = call <vilib>:"Mean PtByPt.vi"("x"=w695, "sample length"="sample length H") -> ("mean"=w694:dbl)  [unwired: 2 in, 1 out]
      "Drehzahl Hinten" <- w694
      n294 = Add(x=w566, y=w565) -> (x+y=w780:dbl)
      n295 = Subtract(x=w563, y=w542) -> (x-y=→"Abweichung":dbl)
      n296 = Divide(x=w621, y=w620) -> (x/y=w633:dbl)
      n297 = Add(x=w544, y=w543) -> (x+y=w703:dbl)
      n298 = Multiply(x=w694, y="Übersetzung H") -> (x*y=→"Wellendrehzahl mit Übersetzung H":dbl)
      n299 = call <vilib>:"Mean PtByPt.vi"("x"=w690, "sample length"="sample length H") -> ("mean"=→"Wellendrehmoment mit Übersetzung  H":dbl)  [unwired: 2 in, 1 out]
      n300 = feedback-in #2(w633) -> ()
      n301 = Divide(x=w703, y="Übersetzung LR") -> (x/y=w546:dbl)
      "Wellendrehmoment mit Übersetzung" <- w546
      n302 = shared-variable "My Computer\\test_1.lvlib\\Drehmoment"(w546) -> ()  [unwired: 1 in, 1 out]
      n303 = Multiply(x=w780, y=w779) -> (x*y=w777:dbl)
      n304 = Divide(x=w546, y=400.0) -> (x/y=w721:dbl)
      n305 = Multiply(x=w777, y="Übersetzung LR") -> (x*y=w606:dbl)
      "Wellendrehzahl mit Übersetzung" <- w606
      n306 = Add(x=w721, y=5.0) -> (x+y=w619:dbl)
      n307 = shared-variable "My Computer\\test_1.lvlib\\Drehzahl"(w606) -> ()  [unwired: 1 in, 1 out]
      n308 = call <vilib>:"Mean PtByPt.vi"("x"=w619, "sample length"="sample length DM") -> ("mean"=w618:dbl)  [unwired: 2 in, 1 out]
      n309 = feedback-in #3(w618) -> ()
      n310 = To Double Precision Float(number=w540) -> (double precision float=→"R":dbl)
      n311 = To Double Precision Float(number=w539) -> (double precision float=→"L":dbl)
    }
    n312 = xnode "Invoke Method"("FPGA VI Reference In"=w2, "error in"=w1) -> ("FPGA VI Reference Out"=w4:refnum<k20>, "error out"=w3:errorcluster)
    n313 = xnode "Invoke Method"("FPGA VI Reference In"=w22, "error in"=w20) -> ("FPGA VI Reference Out"=w14:refnum<k20>, "error out"=w13:errorcluster)
    n314 = xnode "Close FPGA VI Reference"("FPGA VI Reference In"=w4, "error in"=w3) -> ()  [unwired: 1 out]
    n315 = xnode "Close FPGA VI Reference"("FPGA VI Reference In"=w14, "error in"=w13) -> ()  [unwired: 1 out]
  }
